vi "Main_20aa.vi"() -> ()   [LabVIEW 2023]
uses:
  70635ea7-d94a-4e0f-a280-bde64e01a790.vi
  c5597f76-d086-419f-9643-f4e07cdaaf4e.vi
  <vilib>/Comparison/Equal/Equal Functor/Equal Functor.lvclass
panel:
  out "swap value":i32
  out "value":i32
  out "new index":i32
  out "index of element":i32
  out "itteration":i32
  out "remainders":i32[](array[numeric])
  out "end":i32[](array[numeric])
  out "numbers":i32[](array[numeric])
  out "step":i32
  out "Start":i32[](array[numeric])
  out "Before":i32[](array[numeric])
  out "Number":i32
  out "After":i32[](array[numeric])
  out "size(s)":i32
  out "Answer":i32
  in  "Puzzle":string="9688\n470\n-3016\n-5110\n3615\n3862\n6989\n-2605\n-8389\n-3372\n3935\n7241\n-8871\n-2995\n6517\n6929\n3149\n-1876\n4981\n-5525\n-1560\n3851\n-9322\n-2382\n-2710\n7573\n6449\n-1170\n-8779\n-130\n7584\n7483\n60\n7252\n1369\n3120\n9957\n1411\n6218\n-5525\n-8184\n-8998\n1635\n-3127\n-7994\n6051\n-6314\n-8057\n-3556\n6669\n-9474\n-7982\n-1399\n-4627\n-627\n-438\n5027\n-9437\n6378\n-8050\n-718\n8703\n-8195\n2547\n-3543\n3352\n-1818\n2477\n9893\n7017\n-2689\n-8515\n7791\n-1489\n6697\n4362\n-4211\n9311\n-6960\n-452\n-4984\n-9978\n-2261\n2264\n3862\n-2177\n-583\n193\n6958\n-508\n-6946\n-371\n3831\n-8558\n-1592\n3809\n8078\n-1040\n-4311\n590\n5926\n42\n-6730\n8922\n-668\n6372\n9279\n8055\n-5452\n-3522\n-9527\n-9..."
  in  "Example":string="1\n2\n-3\n3\n-2\n0\n4"
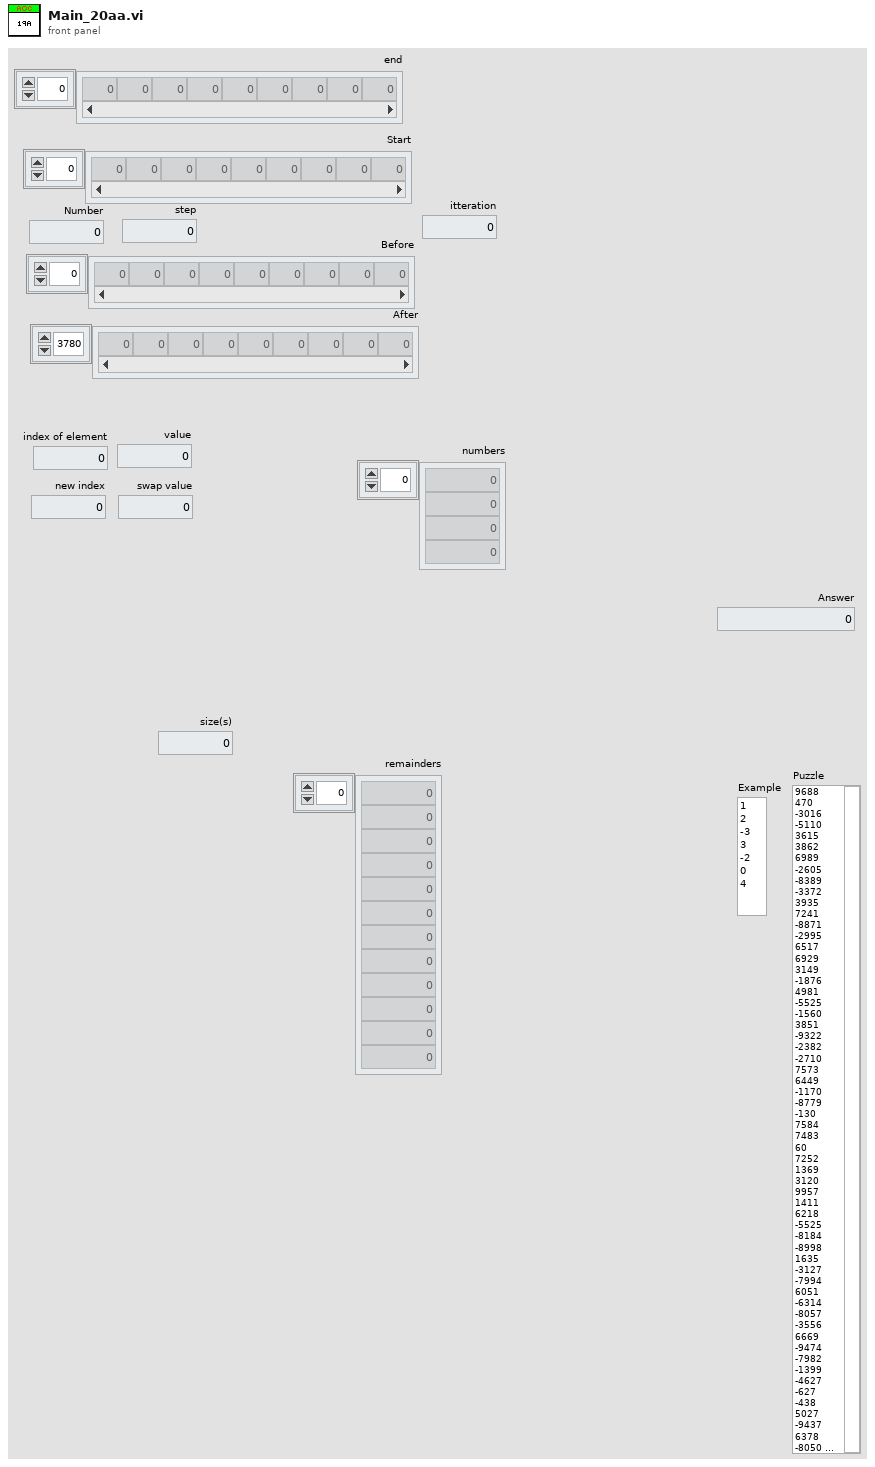
[diagram p1: front panel]
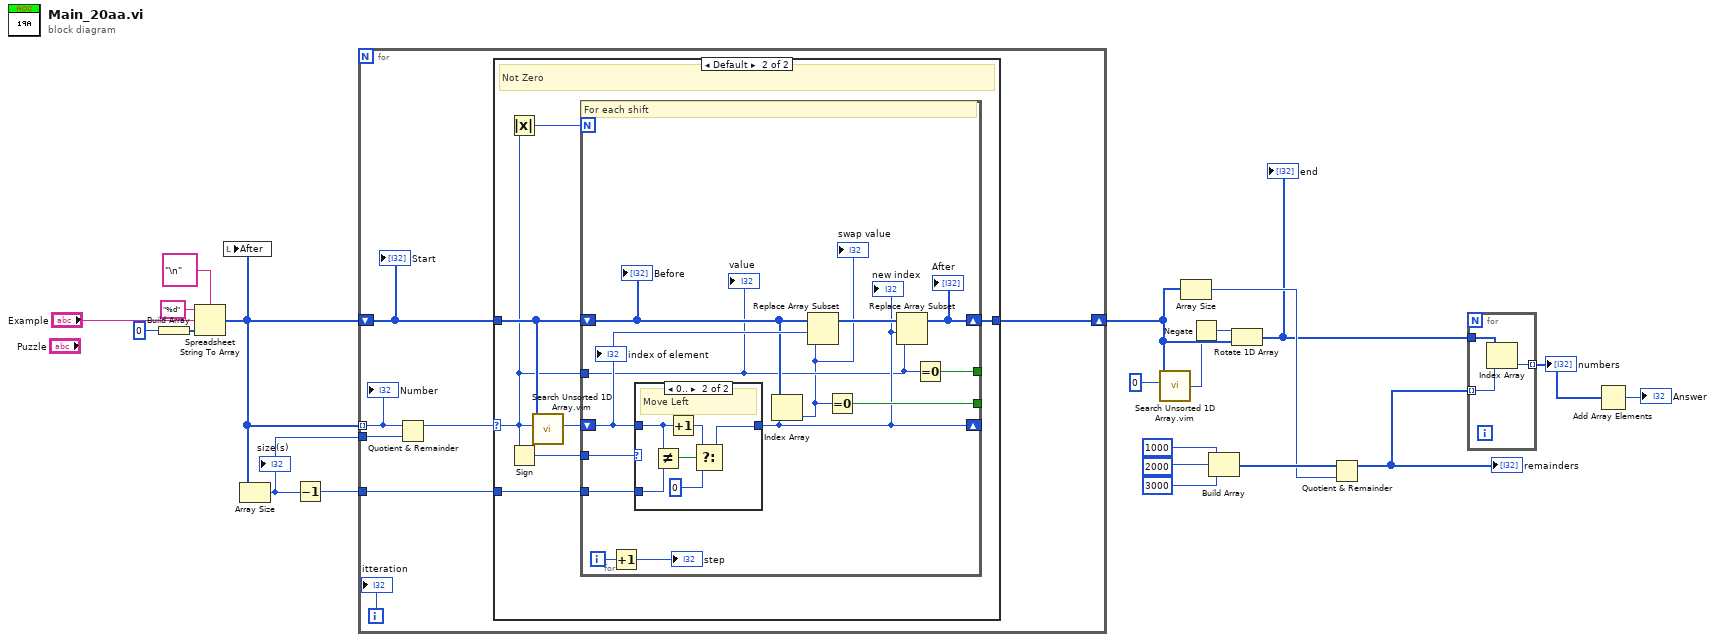
[diagram p0: block diagram]
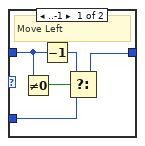
[diagram p3: hidden frame]
diagram:
  n1 = Build Array(0) -> (w21:i32[])
  n2 = Spreadsheet String To Array(delimiter (Tab)="\n", format string="%d", spreadsheet string="Example", array type (2D Dbl)=w21) -> (array=w16:i32[])
  n3 = local write "After"(w16) -> ()
  n4 = Array Size(array=w16) -> (size(s)=w2:i32)
  "size(s)" <- w2
  n5 = Decrement(x=w2) -> (x-1=w17:i32)
  n6 = for {
    tunnel: w16 -> [w23] mode=indexing
    shift-right: [w28] -> w9
    shift-left: w16 -> [w27]
    tunnel: w17 -> [w25]
    tunnel: w2 -> [w22]
    i -> [w26]
    n7 = Quotient & Remainder(x=w23, y=w22) -> (x-y*floor(x/y)=w24:i32)  [unwired: 1 out]
    n8 = case shown="Default" w24 {
      selector: w24 -> [_ w30]
      tunnel: w27 -> [w29 w33]
      tunnel: [w29 w32] -> w28
      tunnel: w25 -> [_ w31]
      frame 0 {
        # "Zero"
      }
      frame Default {
        # "Not Zero"
        n9 = Absolute Value(x=w30) -> (abs(x)=w35:i32)
        n10 = Sign(1:w30) -> (0:w34:i32)
        n11 = call "Search Unsorted 1D Array.vim"("element"=w30, "unsorted 1D array"=w33) -> ("index of element"=w36:i32)  [unwired: 9 in]
        n12 = for {
          N: w35 -> [_]
          shift-right: [w39] -> _
          shift-left: w36 -> [w46]
          tunnel: w34 -> [w49]
          shift-right: [w45] -> w32
          shift-left: w33 -> [w44]
          tunnel: w31 -> [w48]
          tunnel: w30 -> [w38]
          tunnel: [w41] -> _
          tunnel: [w40] -> _
          i -> [w43]
          # "For each shift"
          n13 = Increment(x=w43) -> (x+1=→"step":i32)
          n14 = case shown="0.." w49 {
            tunnel: w46 -> [w53 w56]
            tunnel: w48 -> [w52 w58]
            tunnel: [w51 w60] -> w39
            frame ..-1 {
              # "Move Left"
              n15 = Not Equal To 0?(x=w53) -> (x != 0?=w54:bool)
              n16 = Decrement(x=w53) -> (x-1=w50:i32)
              n17 = Select(t=w50, s=w54, f=w52) -> (s? t:f=w51:i32)
            }
            frame 0.. {
              # "Move Left"
              n18 = Not Equal?(x=w56, y=w58) -> (x != y?=w57:bool)
              n19 = Increment(x=w56) -> (x+1=w59:i32)
              n20 = Select(t=w59, s=w57, f=0) -> (s? t:f=w60:i32)
            }
          }
          "new index" <- w39
          n21 = Index Array(array=w44, index=w39) -> (element=w37:i32)
          "swap value" <- w37
          n22 = Replace Array Subset(array=w44, new element=w37, index=w46) -> (w47:i32[])
          n23 = Equal To 0?(x=w37) -> (x = 0?=w40:bool)
          n24 = Replace Array Subset(array=w47, new element=w38, index=w39) -> (w45:i32[])
          "After" <- w45
          n25 = Equal To 0?(x=w38) -> (x = 0?=w41:bool)
          "Before" <- w44
          "index of element" <- w46
          "value" <- w38
        }
      }
    }
    "Number" <- w23
    "Start" <- w27
    "itteration" <- w26
  }
  n26 = call "Search Unsorted 1D Array.vim"("element"=0 ("Answer 2"), "unsorted 1D array"=w9) -> ("index of element"=w8:i32)  [unwired: 9 in]
  n27 = Array Size(array=w9) -> (size(s)=w10:i32)
  n28 = Negate(x=w8) -> (-x=w7:i32)
  n29 = Build Array(1000 ("Answer 2"), 2000 ("Answer 2"), 3000 ("Answer 2")) -> (w11:i32[])
  n30 = Rotate 1D Array(1:w9, 2:w7) -> (0:w6:i32[])
  "end" <- w6
  n31 = Quotient & Remainder(x=w11, y=w10) -> (x-y*floor(x/y)=w3:i32[])  [unwired: 1 out]
  "remainders" <- w3
  n32 = for {
    tunnel: w6 -> [w63]
    tunnel: w3 -> [w62] mode=indexing
    tunnel: [w61] -> w5 mode=indexing
    n33 = Index Array(array=w63, index=w62) -> (element=w61:i32)
  }
  "numbers" <- w5
  n34 = Add Array Elements(numeric array=w5) -> (sum=→"Answer":i32)
